vi "validate configuration.vi"(8 "error in":errorcluster, 11 "fixed channel configuration in":refnum<class "fixed channel configuration.lvclass">) -> (0 "error out":errorcluster, 3 "fixed channel configuration out":refnum<class "fixed channel configuration.lvclass">)   [LabVIEW 2013, in "fixed channel configuration.lvclass"]
doc: "This function performs validation of the configuration. This function should be safe to call at any point and should not rely on anything in the runtime environment."
uses:
  fixed channel configuration.lvclass
  <vilib>/NI/Tag Bus Module Framework/module configuration/TBM module configuration.lvclass
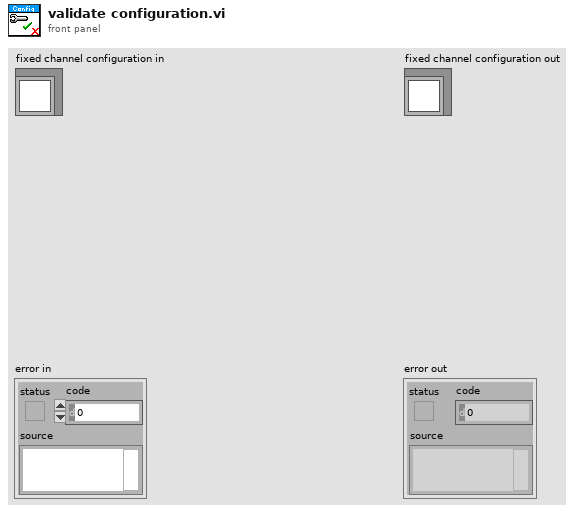
[diagram p1: front panel]
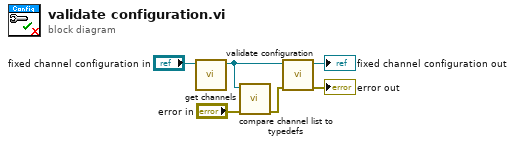
[diagram p0: block diagram]
diagram:
  n1 = call-dynamic "get channels.vi"("fixed channel configuration in"="fixed channel configuration in") -> ("fixed channel configuration out"=w1:refnum<class "fixed channel configuration.lvclass">)  [unwired: 9 in, 1 out]
  n2 = call "compare channel list to typedefs.vi"("error in"="error in", "fixed channel configuration"=w1) -> ("error out"=w3:errorcluster)  [unwired: 8 in, 1 out]
  n3 = call-parent "validate configuration.vi"("error in"=w3, "configuration in"=w1) -> ("error out"=→"error out":errorcluster, "configuration out"=→"fixed channel configuration out":refnum<class "fixed channel configuration.lvclass">)  [unwired: 8 in]
